vi "set_linear_intensity.vi"(8 "error in (no error)":errorcluster, 10 "power slider in":cluster{dbl, dbl}, 11 "number of frames":i32) -> (0 "error out":errorcluster, 3 "amplitude out":u16[](array[numeric]))   [LabVIEW 2010, in "TrajectoryMH100122AODRAPS.lvclass"]
uses:
  TrajectoryMH100122AODRAPS.lvclass
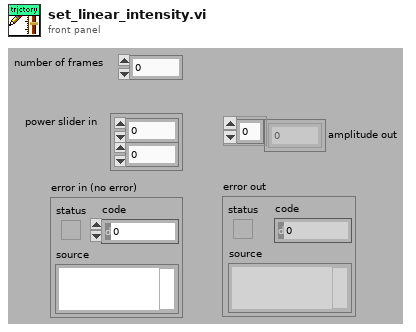
[diagram p1: front panel]
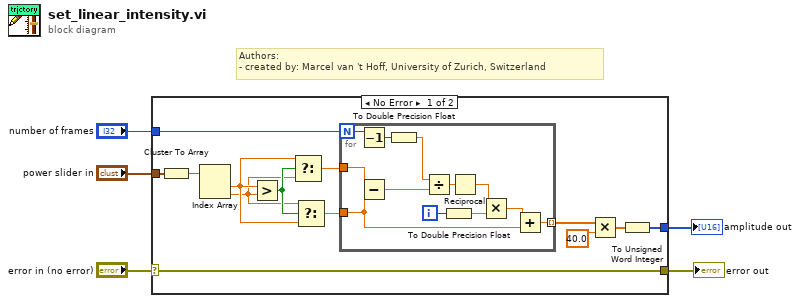
[diagram p0: block diagram]
diagram:
  # "Authors: \n- created by: Marcel van 't Hoff, University of Zurich, Switzerland"
  n1 = case shown="No Error" "error in (no error)" {
    selector: "error in (no error)" -> [w6 w31]
    tunnel: [w18 _] -> w5
    tunnel: "number of frames" -> [w9 _]
    tunnel: "power slider in" -> [w7 _]
    tunnel: [w6 w31] -> w1
    frame No Error {
      n2 = Cluster To Array(cluster=w7) -> (array=w8:dbl[])
      n3 = Index Array(array=w8) -> (element #1=w11:dbl, element #2=w10:dbl)  [unwired: 2 in]
      n4 = Greater?(x=w11, y=w10) -> (0:w12:bool)
      n5 = Select(t=w11, s=w12, f=w10) -> (s? t:f=w13:dbl)
      n6 = Select(t=w10, s=w12, f=w11) -> (s? t:f=w14:dbl)
      n7 = for {
        N: w9 -> [w29]
        tunnel: w13 -> [w30]
        tunnel: w14 -> [w19]
        tunnel: [w20] -> w15 mode=indexing
        i -> [w24]
        n8 = Decrement(x=w29) -> (x-1=w21:i32)
        n9 = Subtract(x=w30, y=w19) -> (x-y=w27:dbl)
        n10 = To Double Precision Float(number=w21) -> (double precision float=w26:dbl)
        n11 = Divide(x=w26, y=w27) -> (x/y=w28:dbl)
        n12 = To Double Precision Float(number=w24) -> (double precision float=w23:dbl)
        n13 = Reciprocal(x=w28) -> (1/x=w25:dbl)
        n14 = Multiply(x=w25, y=w23) -> (x*y=w22:dbl)
        n15 = Add(x=w22, y=w19) -> (x+y=w20:dbl)
      }
      n16 = Multiply(x=w15, y=40.0 ("s? t:f")) -> (x*y=w17:dbl[])
      n17 = To Unsigned Word Integer(number=w17) -> (unsigned 16bit integer=w18:u16[])
    }
    frame Error {
    }
  }
  "amplitude out" <- w5
  "error out" <- w1
